vi "Zadanie 1.vi"() -> ()   [LabVIEW 2020]
panel:
  in  "Zmien  cosinusa":u16(ring) items=["1", "2", "3", "4", "5"]
  in  "Zmien sinusa":u16(ring) items=["1", "2", "3", "4", "5"]
  in  "Zmien kolor cos":u32(colorbox)
  in  "Zmien kolor sin":u32(colorbox)
  in  "Nazwa cosinus":string
  in  "Nazwa sinusa":string
  in  "Zniknij legendê":bool
  in  "stop":bool
  in  "Zniknij wykres":bool
  in  "N 2":i32
  in  "Amplituda 2":dbl
  in  "Faza 2":dbl
  in  "k 2":dbl
  out "XY Graph":cluster{i32[], "Array":dbl[]}[](graph)
  in  "k":dbl
  in  "N":i32
  in  "Faza":dbl
  in  "Amplituda":dbl
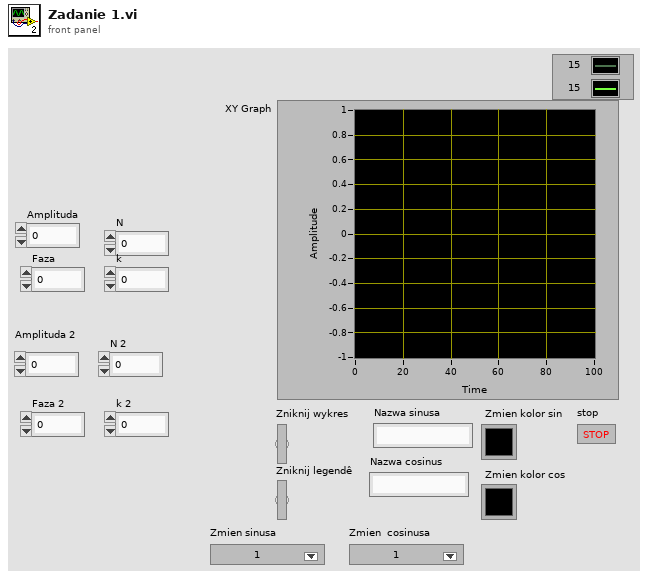
[diagram p1: front panel]
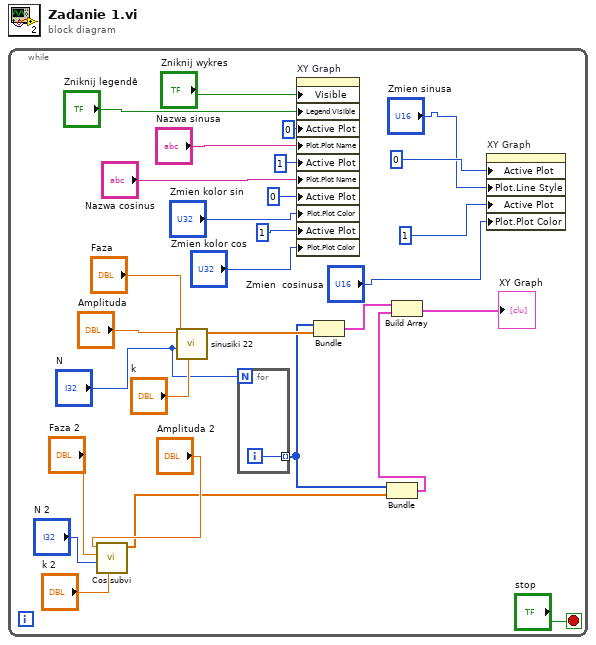
[diagram p0: block diagram]
diagram:
  n1 = while {
    stop <- "stop" stop-if-true
    n2 = call "Cos subvi.vi"("k in"="k 2", "N in"="N 2", "Faza in"="Faza 2", "Amplituda in"="Amplituda 2") -> ("Array"=w20:dbl[])  [unwired: 7 in]
    n3 = call "sinusiki 22.vi"("k"="k", "N"="N", "Faza"="Faza", "Amplituda"="Amplituda") -> ("Array"=w24:dbl[])  [unwired: 7 in]
    n4 = for {
      N: "N" -> [_]
      tunnel: [w30] -> w17 mode=indexing
      i -> [w30]
    }
    n5 = property on="XY Graph" class="XYGraph (strict)"("Visible"="Zniknij wykres", "Legend Visible"="Zniknij legendê", "Active Plot"=0, "Plot.Plot Name"="Nazwa sinusa", "Active Plot"=1, "Plot.Plot Name"="Nazwa cosinus", "Active Plot"=0, "Plot.Plot Color"="Zmien kolor sin", "Active Plot"=1, "Plot.Plot Color"="Zmien kolor cos") -> ()  [unwired: 2 in, 2 out]
    n6 = Bundle(w17, "Array"=w24) -> (w25:cluster{i32[], "Array":dbl[]})  [unwired: 1 in]
    n7 = Bundle(w17, "Array"=w20) -> (w19:cluster{i32[], "Array":dbl[]})  [unwired: 1 in]
    n8 = Build Array(w25, w19) -> (→"XY Graph":cluster{i32[], "Array":dbl[]}[])
    n9 = property on="XY Graph" class="XYGraph (strict)"("Active Plot"=0, "Plot.Line Style"="Zmien sinusa", "Active Plot"=1, "Plot.Plot Color"="Zmien  cosinusa") -> ()  [unwired: 2 in, 2 out]
  }
